vi "Actual Pressure SI.vi"(8 "Error In":errorcluster, 11 "VISA resource name":refnum<visa-resource-name>) -> (0 "Error Out":errorcluster, 1 "Pressure":dbl[unit], 3 "dup VISA resource name":refnum<visa-resource-name>)   [LabVIEW 2011, in "MGC647C.lvlib"]
doc: "Retrun actual pressure in SI unit.\n\n<b>Remember:</b> 1 Torr = 133.3 Pa and 1 mBar = 1 hPa."
uses:
  <instrlib>/MGC647C/MGC647C.lvlib
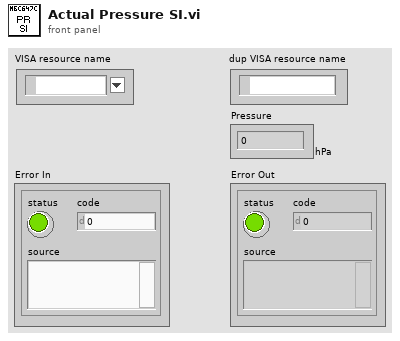
[diagram p1: front panel]
types:
  T1 = enum16{"1.0000 mTorr", "10.000 mTorr", "100.00 mTorr", "1000.0 mTorr", "1.0000 Torr", "10.000 Torr", "100.00 Torr", "1000.0 Torr", "1.0000 kTorr", "10.000 kTorr", "100.00 kTorr", "1.0000 µBar", "10.000 µBar", "100.00 µBar", "1000.0 µBar", "1.0000 mBar", "10.000 mBar", "100.00 mBar", "1000.0 mBar", "1.0000 Bar", "10.000 Bar", "100.00 Bar", "1.0000 Pa", "10.000 Pa", "100.00 Pa", "1.0000 kPa", "10.000 kPa", "100.00 kPa", "1000.0 kPa"}
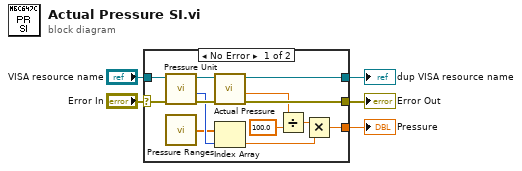
[diagram p0: block diagram]
diagram:
  n1 = case shown="No Error" "Error In" {
    selector: "Error In" -> [w17 w20]
    tunnel: "VISA resource name" -> [w18 w19]
    tunnel: [w14 w19] -> w4
    tunnel: [w13 w20] -> w3
    tunnel: [w7 _] -> w1
    frame No Error {
      n2 = call <instrlib>:"Pressure Unit.vi"("Error In"=w17, "VISA resource name"=w18) -> ("Error Out"=w15:errorcluster, "Unit out"=w12:T1, "dup VISA resource name"=w16:refnum<visa-resource-name>)  [unwired: 7 in]
      n3 = call <instrlib>:"Pressure Ranges.vi"() -> ("Pressure Ranges"=w6:dbl[unit][])
      n4 = call <instrlib>:"Actual Pressure.vi"("Error In"=w15, "VISA resource name"=w16) -> ("Error Out"=w13:errorcluster, "Actual Pressure"=w11:dbl, "dup VISA resource name"=w14:refnum<visa-resource-name>)  [unwired: 7 in]
      n5 = Index Array(array=w6, index=w12) -> (element=w8:dbl[unit])
      n6 = Divide(x=w11, y=100.0) -> (x/y=w9:dbl)
      n7 = Multiply(x=w9, y=w8) -> (x*y=w7:dbl[unit])
    }
    frame Error {
    }
  }
  "dup VISA resource name" <- w4
  "Error Out" <- w3
  "Pressure" <- w1
